vi "Conv_Radians_Deg.vi"(10 "Radians":dbl) -> (2 "Degrees":dbl)   [LabVIEW 2019, in "Trajectory_Library.lvlib"]
doc: "Convert Radians to Degrees"
uses:
  Trajectory_Library.lvlib
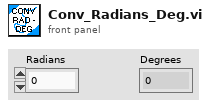
[diagram p1: front panel]
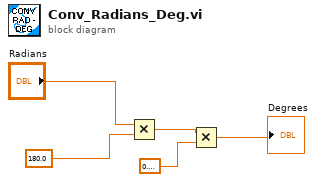
[diagram p0: block diagram]
diagram:
  n1 = Multiply(x="Radians", y=180.0) -> (x*y=w3:dbl)
  n2 = Multiply(x=w3, y=0.3183098861837907) -> (x*y=→"Degrees":dbl)
